vi "Main VI.vi"() -> ()   [LabVIEW 2019]
panel:
  in  "Validate Authentification":bool
  in  "Confirm Selected Mode":bool
  out "AUTHENFICATION FEEDBACK":string
  in  "Stop Program":bool
  in  "Reset":bool
  in  "New Learning ?":bool
  in  "Conversion Mode":string(combo)
  out "LOGIN&PASSWORD":bool
  in  "Password":string
  in  "Name":string
  in  "First Name":string
  # "Get started by fill inputs bellow to access to the BEST APPLICATION ever."
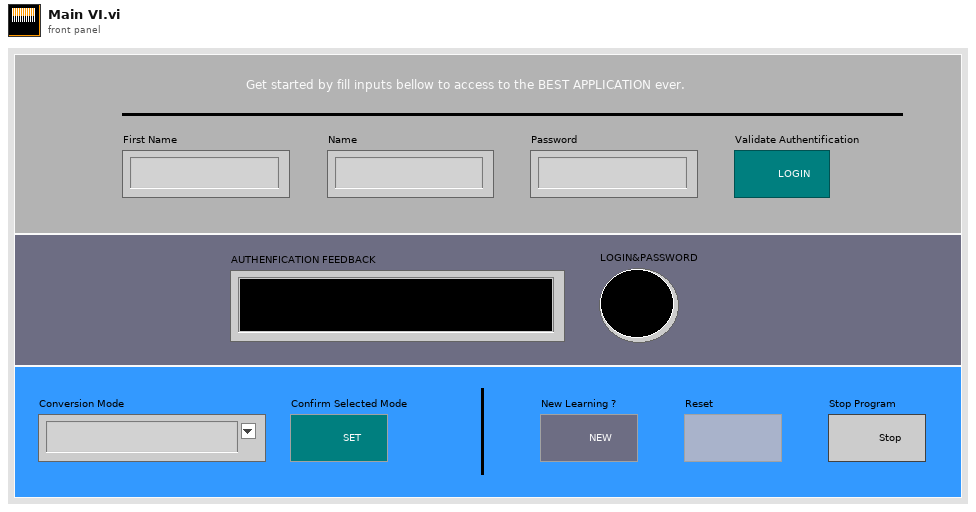
[diagram p1: front panel]
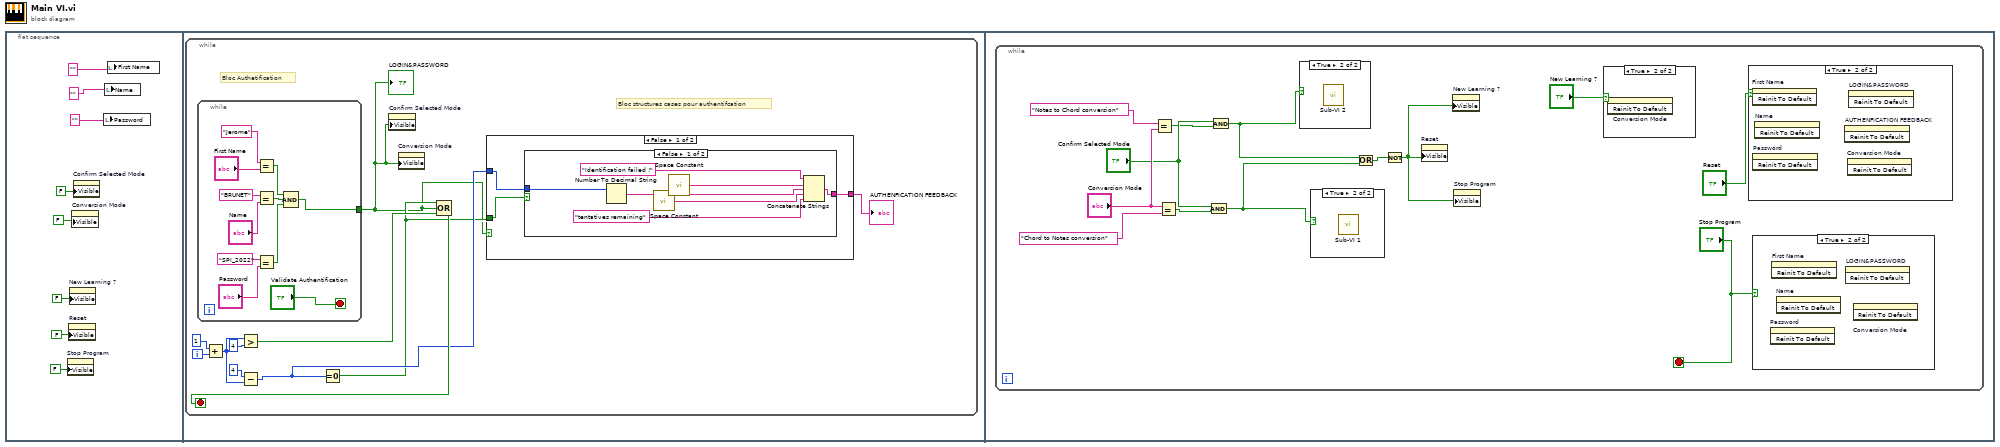
[diagram p0: block diagram]
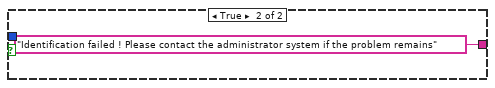
[diagram p2: hidden frame]
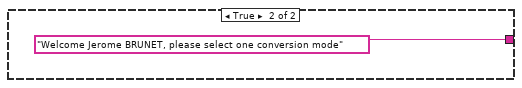
[diagram p3: hidden frame]
diagram:
  n1 = flat-sequence {
    frame #0 {
      n2 = property on="Stop Program" class="Bool"("Visible"=FALSE) -> ()  [unwired: 2 in, 2 out]
      n3 = property on="Reset" class="Bool"("Visible"=FALSE) -> ()  [unwired: 2 in, 2 out]
      n4 = property on="New Learning ?" class="Bool"("Visible"=FALSE) -> ()  [unwired: 2 in, 2 out]
      n5 = property on="Conversion Mode" class="CmbBox"("Visible"=FALSE) -> ()  [unwired: 2 in, 2 out]
      n6 = property on="Confirm Selected Mode" class="Bool"("Visible"=FALSE) -> ()  [unwired: 2 in, 2 out]
      n7 = local write "Password"("") -> ()
      n8 = local write "Name"("") -> ()
      n9 = local write "First Name"("") -> ()
    }
    frame #1 {
      n10 = while {
        i -> [w18]
        stop <- w19 stop-if-true
        # "Bloc structures cases pour authentifcation"
        # "Bloc Authetification"
        n11 = while {
          tunnel: [w33] -> w9
          stop <- "Validate Authentification" stop-if-true
          n12 = Equal?(x="Jerome", y="First Name") -> (x = y?=w36:bool)
          n13 = Equal?(x="BRUNET", y="Name") -> (x = y?=w35:bool)
          n14 = Equal?(x="SPI_2022", y="Password") -> (x = y?=w34:bool)
          n15 = Compound Arithmetic op=AND ("Opérateur arithmétique")(w36, w35, w34) -> (w33:bool)
        }
        "LOGIN&PASSWORD" <- w9
        n16 = Add(x=1, y=w18) -> (x+y=w16:i32)
        n17 = Greater?(x=w16, y=4) -> (0:w13:bool)
        n18 = Subtract(x=4, y=w16) -> (x-y=w12:i32)
        n19 = Equal To 0?(x=w12) -> (x = 0?=w10:bool)
        n20 = property on="Confirm Selected Mode" class="Bool"("Visible"=w9) -> ()  [unwired: 2 in, 2 out]
        n21 = property on="Conversion Mode" class="CmbBox"("Visible"=w9) -> ()  [unwired: 2 in, 2 out]
        n22 = Compound Arithmetic op=OR ("Opérateur arithmétique")(w10, w9, w13) -> (w19:bool)
        n23 = case shown="False" w9 {
          tunnel: w12 -> [w22 _]
          tunnel: [w21 "Welcome Jerome BRUNET, please select one conversion mode"] -> w11
          tunnel: w10 -> [w20 _]
          frame False {
            n24 = case shown="False" w20 {
              tunnel: w22 -> [w29 _]
              tunnel: [w28 "Identification failed ! Please contact the administrator system if the problem remains"] -> w21
              frame False {
                n25 = Number To Decimal String(number=w29) -> (decimal integer string=w25:string)  [unwired: 1 in]
                n26 = call <vilib>:"Space Constant.vi"() -> ("String"=w24:string)
                n27 = call <vilib>:"Space Constant.vi"() -> ("String"=w26:string)
                n28 = Concatenate Strings("Identification failed !", w26, w25, w24, "tentatives remaining") -> (w28:string)
              }
              frame True {
              }
            }
          }
          frame True {
          }
        }
        "AUTHENFICATION FEEDBACK" <- w11
      }
    }
    frame #2 {
      n29 = while {
        stop <- "Stop Program" stop-if-true
        n30 = Equal?(x="Notes to Chord conversion", y="Conversion Mode") -> (x = y?=w53:bool)
        n31 = Equal?(x="Conversion Mode", y="Chord to Notes conversion") -> (x = y?=w52:bool)
        n32 = And(x="Confirm Selected Mode", y=w52) -> (x .and. y?=w43:bool)
        n33 = And(x="Confirm Selected Mode", y=w53) -> (x .and. y?=w44:bool)
        n34 = case shown="True" w44 {
          frame False {
          }
          frame True {
            n35 = call "Sub-VI 2.vi"() -> ()  [unwired: 27 in, 1 out]
          }
        }
        n36 = case shown="True" w43 {
          frame False {
          }
          frame True {
            n37 = call "Sub-VI 1.vi"() -> ()  [unwired: 9 in, 19 out]
          }
        }
        n38 = Or(x=w44, y=w43) -> (x .or. y?=w51:bool)
        n39 = Not(x=w51) -> (.not. x?=w50:bool)
        n40 = property on="Reset" class="Bool"("Visible"=w50) -> ()  [unwired: 2 in, 2 out]
        n41 = property on="New Learning ?" class="Bool"("Visible"=w50) -> ()  [unwired: 2 in, 2 out]
        n42 = property on="Stop Program" class="Bool"("Visible"=w50) -> ()  [unwired: 2 in, 2 out]
        n43 = case shown="True" "New Learning ?" {
          frame False {
          }
          frame True {
            n44 = invoke on="Conversion Mode" class="CmbBox" method="Reinit To Default"() -> ()  [unwired: 3 in, 3 out]
          }
        }
        n45 = case shown="True" "Reset" {
          frame False {
          }
          frame True {
            n46 = invoke on="First Name" class="Str" method="Reinit To Default"() -> ()  [unwired: 3 in, 3 out]
            n47 = invoke on="Password" class="Str" method="Reinit To Default"() -> ()  [unwired: 3 in, 3 out]
            n48 = invoke on="Name" class="Str" method="Reinit To Default"() -> ()  [unwired: 3 in, 3 out]
            n49 = invoke on="AUTHENFICATION FEEDBACK" class="Str" method="Reinit To Default"() -> ()  [unwired: 3 in, 3 out]
            n50 = invoke on="Conversion Mode" class="CmbBox" method="Reinit To Default"() -> ()  [unwired: 3 in, 3 out]
            n51 = invoke on="LOGIN&PASSWORD" class="Bool (strict)" method="Reinit To Default"() -> ()  [unwired: 3 in, 3 out]
          }
        }
        n52 = case shown="True" "Stop Program" {
          frame False {
          }
          frame True {
            n53 = invoke on="Password" class="Str" method="Reinit To Default"() -> ()  [unwired: 3 in, 3 out]
            n54 = invoke on="First Name" class="Str" method="Reinit To Default"() -> ()  [unwired: 3 in, 3 out]
            n55 = invoke on="Name" class="Str" method="Reinit To Default"() -> ()  [unwired: 3 in, 3 out]
            n56 = invoke on="LOGIN&PASSWORD" class="Bool (strict)" method="Reinit To Default"() -> ()  [unwired: 3 in, 3 out]
            n57 = invoke on="Conversion Mode" class="CmbBox" method="Reinit To Default"() -> ()  [unwired: 3 in, 3 out]
          }
        }
      }
    }
  }
